vi "_Get RT Lens Configuration.vi"(5 "Name":string, 7 "Channel #":u8) -> (1 "Config Row#":i32, 3 "Lens Configuration":T1)   [LabVIEW 2012]
uses:
  Type/_RT Configuration 2.ctl
  _RT Global.vi
panel:
  # "Get lens properties from a configuration table by ch# or name"
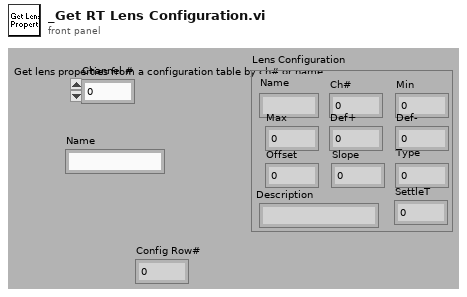
[diagram p1: front panel]
types:
  T1 = typedef "_RT Configuration 2.ctl" = cluster{"Name":string, "Ch#":u8, "Min":dbl, "Max":dbl, "Def+":dbl, "Def-":dbl, "Offset":dbl, "Slope":dbl, "Type":u8, "Description":string, "SettleT":dbl}
  T2 = typedef "_RT Instrument 2.ctl" = cluster{"Table":T1[], "Instrument":string[]}
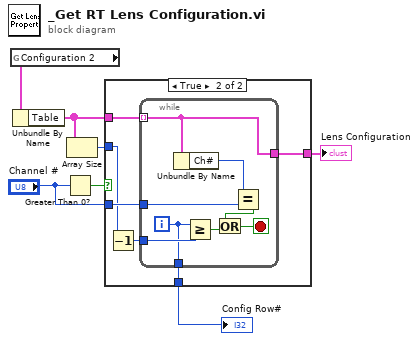
[diagram p0: block diagram]
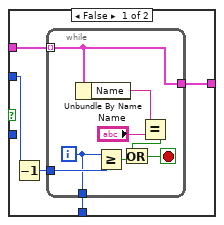
[diagram p2: hidden frame]
diagram:
  n1 = global read "_RT Global.vi" "Configuration 2"() -> (w1:T2)
  n2 = Unbundle By Name(w1) -> ("Table"=w5:T1[])
  n3 = Greater Than 0?(x="Channel #") -> (x > 0?=w7:bool)
  n4 = Array Size(array=w5) -> (size(s)=w4:i32)
  n5 = case shown="True" w7 {
    tunnel: w5 -> [w11 w26]
    tunnel: [w12 w25] -> w3
    tunnel: "Channel #" -> [_ w24]
    tunnel: w4 -> [w10 w23]
    tunnel: [w8 w21] -> w2
    frame False {
      n6 = Decrement(x=w10) -> (x-1=w9:i32)
      n7 = while {
        tunnel: w11 -> [w16] mode=indexing
        tunnel: [w16] -> w12
        tunnel: w9 -> [w17]
        tunnel: [w13] -> w8
        i -> [w13]
        stop <- w20 stop-if-true
        n8 = Unbundle By Name(w16) -> ("Name"=w15:string)
        n9 = Greater Or Equal?(x=w13, y=w17) -> (x >= y?=w18:bool)
        n10 = Equal?(x=w15, y="Name") -> (x = y?=w19:bool)
        n11 = Or(x=w19, y=w18) -> (x .or. y?=w20:bool)
      }
    }
    frame True {
      n12 = Decrement(x=w23) -> (x-1=w22:i32)
      n13 = while {
        tunnel: w26 -> [w29] mode=indexing
        tunnel: [w29] -> w25
        tunnel: w24 -> [w34]
        tunnel: w22 -> [w30]
        tunnel: [w27] -> w21
        i -> [w27]
        stop <- w33 stop-if-true
        n14 = Unbundle By Name(w29) -> ("Ch#"=w28:u8)
        n15 = Greater Or Equal?(x=w27, y=w30) -> (x >= y?=w31:bool)
        n16 = Equal?(x=w28, y=w34) -> (x = y?=w32:bool)
        n17 = Or(x=w32, y=w31) -> (x .or. y?=w33:bool)
      }
    }
  }
  "Lens Configuration" <- w3
  "Config Row#" <- w2
